vi "Drive Displacement Y.vi"(3 "Error In":errorcluster, 4 "Boolean":bool, 5 "Distance to Drive":dbl) -> (0 "Error Out":errorcluster)   [LabVIEW 2018]
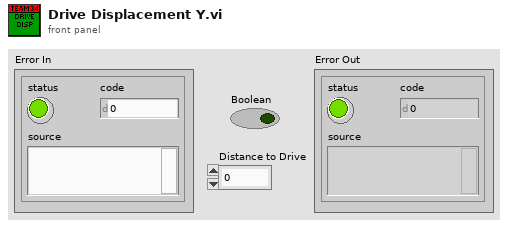
[diagram p1: front panel]
types:
  T1 = cluster{"Velocity X":dbl, "Velocity Y":dbl, "Velocity Z":dbl, "Displacement X":dbl, "Displacement Y":dbl, "Displacement Z":dbl}
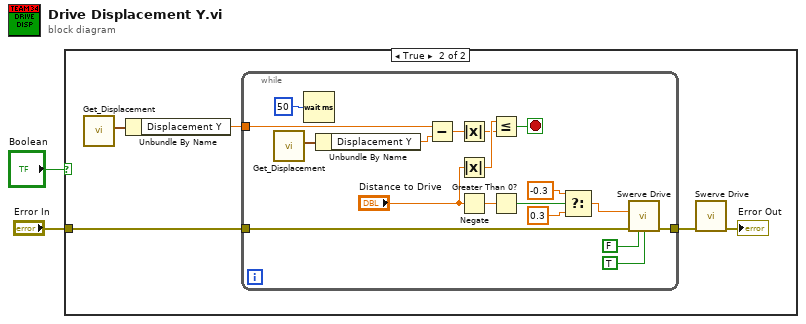
[diagram p0: block diagram]
diagram:
  n1 = case shown="True" "Boolean" {
    tunnel: "Error In" -> [_ w3]
    frame False {
    }
    frame True {
      n2 = call <vilib>:"Get_Displacement.vi"() -> ("Displacement"=w5:T1)  [unwired: 11 in]
      n3 = Unbundle By Name(w5) -> ("Displacement Y"=w6:dbl)
      n4 = while {
        tunnel: [w25] -> w7
        tunnel: w6 -> [w11]
        tunnel: w3 -> [w8]
        stop <- w14 stop-if-true
        n5 = call <vilib>:"Get_Displacement.vi"() -> ("Displacement"=w9:T1)  [unwired: 11 in]
        n6 = Wait (ms)(milliseconds to wait=u32 50) -> ()  [unwired: 1 out]
        n7 = Unbundle By Name(w9) -> ("Displacement Y"=w10:dbl)
        n8 = Subtract(x=w11, y=w10) -> (x-y=w12:dbl)
        n9 = Absolute Value(x=w12) -> (abs(x)=w13:dbl)
        n10 = Absolute Value(x="Distance to Drive") -> (abs(x)=w15:dbl)
        n11 = Negate(x="Distance to Drive") -> (-x=w17:dbl)
        n12 = Less Or Equal?(x=w15, y=w13) -> (x <= y?=w14:bool)
        n13 = Greater Than 0?(x=w17) -> (x > 0?=w20:bool)
        n14 = Select(t=-0.3 ("X"), s=w20, f=0.3 ("X")) -> (s? t:f=w19:dbl)
        n15 = call "Swerve Drive.vi"("Y"=w19, "Error In"=w8, "Robot Centric?"=FALSE, "Autonomous?"=TRUE) -> ("Error Out"=w25:errorcluster)  [unwired: 7 in, 4 out]
      }
      n16 = call "Swerve Drive.vi"("Error In"=w7) -> ("Error Out"=→"Error Out":errorcluster)  [unwired: 10 in, 4 out]
    }
  }
